vi "Close.vi"(8 "error in (no error)":errorcluster, 11 "Prototype Measurement in":refnum<class "Prototype Measurement.lvclass">) -> (0 "error out":errorcluster, 3 "Prototype Measurement out":refnum<class "Prototype Measurement.lvclass">)   [LabVIEW 2016]
uses:
  Measurement/Prototype Measurement.lvclass
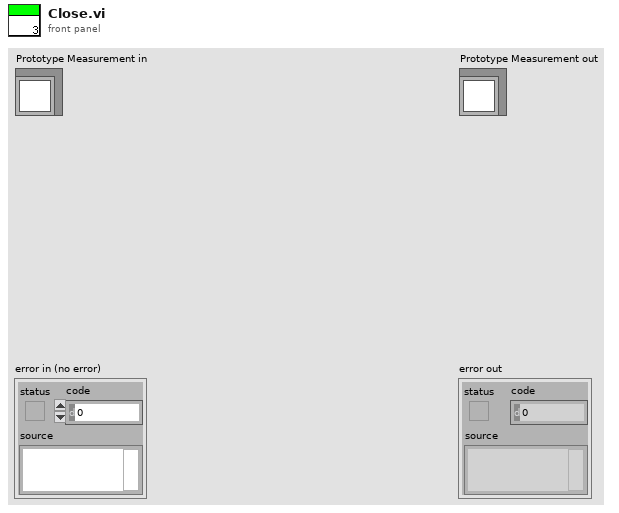
[diagram p1: front panel]
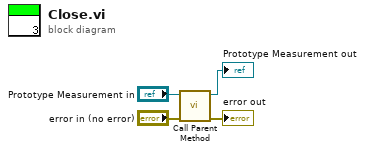
[diagram p0: block diagram]
diagram:
  n1 = call-parent "Call Parent Method"("error in (no error)"="error in (no error)", "Measurement in"="Prototype Measurement in") -> ("error out"=→"error out":errorcluster, "Measurement out"=→"Prototype Measurement out":refnum<class "Prototype Measurement.lvclass">)  [unwired: 8 in]
